vi "DepthSense Connect Callback.vi"(4 "User Parameter":variant, 6 "Control Ref":refnum<k24>, 7 "Event Common Data":T1) -> ()   [LabVIEW 2011]
uses:
  C:/Users/Behavior Room/Desktop/Kinect Mouse/DepthSense/FunctionPointerProxy/FunctionPointerProxy/bin/Release/FunctionPointerProxy.dll
  FunctionPointerProxy/FunctionPointerProxy/bin/Release/FunctionPointerProxy.dll
  DepthSense Global Status.vi
  <userlib>/libOptrima-2-3/libOptrima-2-3.lvlib
panel:
  out "error out":errorcluster
  out "camera version":string
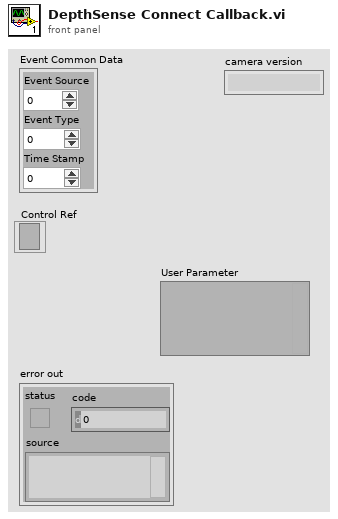
[diagram p1: front panel]
types:
  T1 = cluster{"Event Source":i32, "Event Type":u32, "Time Stamp":u32}
  T2 = cluster{"Camera Version":string, "Image Height":i32, "Image Width":i32, "Minimum Framerate":i32, "Maximum Framerate":i32, "Framerate":i32, "Close Mode":bool, "Denoising":bool, "Leakage Algorithm":bool, "Anti-Aliasing":bool, "Camera Status":i32, "API Version":string, "Light Intensity":i32, "Confidence Threshold":u16, "Range":sgl}
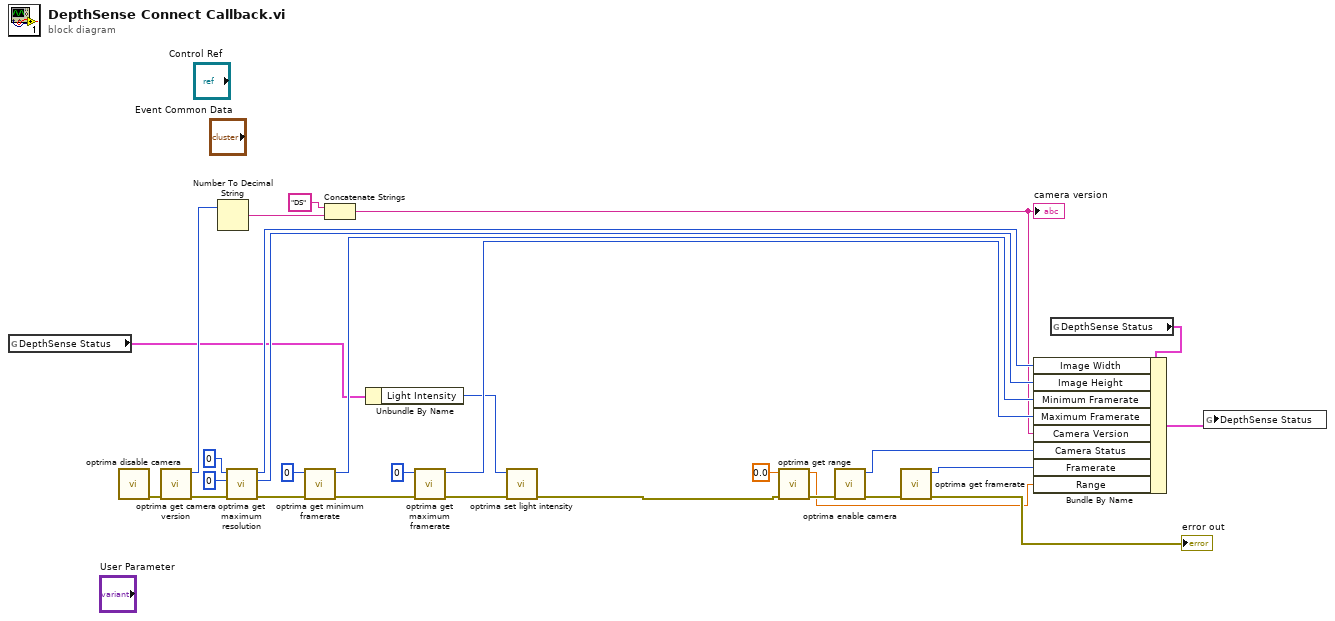
[diagram p0: block diagram]
diagram:
  n1 = global read "DepthSense Global Status.vi" "DepthSense Status"() -> (w9:T2)
  n2 = call <userlib>:"optrima disable camera.vi"() -> ("error out"=w29:errorcluster)  [unwired: 10 in, 1 out]
  n3 = call <userlib>:"optrima get camera version.vi"("error in (no error)"=w29) -> ("error out"=w19:errorcluster, "version out"=w28:u32)  [unwired: 8 in, 1 out]
  n4 = Number To Decimal String(number=w28) -> (decimal integer string=w27:string)  [unwired: 1 in]
  n5 = call <userlib>:"optrima get maximum resolution.vi"("error in (no error)"=w19, "rows"=u32 0, "columns"=u32 0) -> ("error out"=w23:errorcluster, "rows out"=w17:u32, "columns out"=w18:u32)  [unwired: 5 in, 1 out]
  n6 = call <userlib>:"optrima get minimum framerate.vi"("error in (no error)"=w23, "min_framerate"=u32 0) -> ("error out"=w21:errorcluster, "min_framerate out"=w16:u32)  [unwired: 7 in, 1 out]
  n7 = Concatenate Strings("DS" ("string"), w27) -> (w14:string)
  "camera version" <- w14
  n8 = Unbundle By Name(w9) -> ("Light Intensity"=w11:i32)
  n9 = call <userlib>:"optrima get maximum framerate.vi"("error in (no error)"=w21, "max_framerate"=u32 0) -> ("error out"=w13:errorcluster, "max_framerate out"=w15:u32)  [unwired: 7 in, 1 out]
  n10 = call <userlib>:"optrima set light intensity.vi"("error in (no error)"=w13, "intensity_percentage"=w11) -> ("error out"=w1:errorcluster)  [unwired: 8 in, 1 out]
  n11 = call <userlib>:"optrima get range.vi"("error in (no error)"=w1, "range_meters"=sgl 0.0) -> ("error out"=w4:errorcluster, "range_meters out"=w2:sgl)  [unwired: 7 in, 1 out]
  n12 = call <userlib>:"optrima enable camera.vi"("error in (no error)"=w4) -> ("error out"=w12:errorcluster, "function return"=w5:u32)  [unwired: 9 in]
  n13 = call <userlib>:"optrima get framerate.vi"("error in (no error)"=w12) -> ("error out"=→"error out":errorcluster, "framerate out"=w10:u32)  [unwired: 8 in, 1 out]
  n14 = global read "DepthSense Global Status.vi" "DepthSense Status"() -> (w7:T2)
  n15 = Bundle By Name(cluster=w7, "Image Width"=w18, "Image Height"=w17, "Minimum Framerate"=w16, "Maximum Framerate"=w15, "Camera Version"=w14, "Camera Status"=w5, "Framerate"=w10, "Range"=w2) -> (w8:T2)
  n16 = global write "DepthSense Global Status.vi" "DepthSense Status"(w8) -> ()
